vi "Write Command.vi"(8 "error in (no error)":errorcluster, 9 "Command":string, 11 "VISA resource name":refnum<visa-resource-name>) -> (0 "error out":errorcluster, 3 "VISA resource name out":refnum<visa-resource-name>)   [LabVIEW 2020, in "Rohde&Schwarz CMP LR WPAN Measurement.lvlib"]
doc: "This VI sends a SCPI command to the instrument. Do not use this VI for queries (SCPI commands ending with the questiomark e.g. OUTPUT:STATE? )\nFor queries, use one of the following VIs:\n- <b>Query ViBoolean.vi</b>\n- <b>Query ViInt32.vi</b>\n- <b>Query ViReal64.vi</b>\n- <b>Query ViString.vi</b>\n- <b>Query with OPC sync.vi</b>"
uses:
  <instrlib>/Rohde&Schwarz CMP LR WPAN Measurement/Rohde&Schwarz CMP LR WPAN Measurement.lvlib
  <instrlib>/Rohde&Schwarz CMP LR WPAN Measurement/Private/rsidr_core.llb/rsidr_core.lvlib
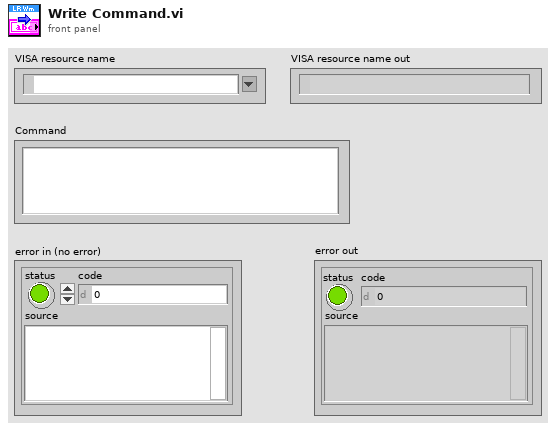
[diagram p1: front panel]
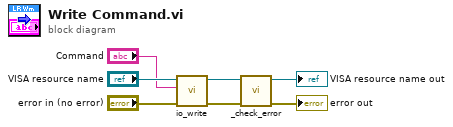
[diagram p0: block diagram]
diagram:
  n1 = call <instrlib>:"io_write.vi"("error in"="error in (no error)", "write buffer"="Command", "VISA resource name"="VISA resource name") -> ("error out"=w5:errorcluster, "VISA resource name out"=w4:refnum<visa-resource-name>)  [unwired: 7 in]
  n2 = call <instrlib>:"_check_error.vi"("error in (no error)"=w5, "VISA resource name"=w4) -> ("error out"=→"error out":errorcluster, "VISA resource name out"=→"VISA resource name out":refnum<visa-resource-name>)  [unwired: 8 in]
